vi "Exercise 5.2.vi"() -> ()   [LabVIEW 2020]
panel:
  in  "Control 2":dbl
  out "Waveform Chart 2":dbl(graph)
  in  "Master Stop":bool
  out "Waveform Chart 1":dbl(graph)
  in  "Control 1":dbl
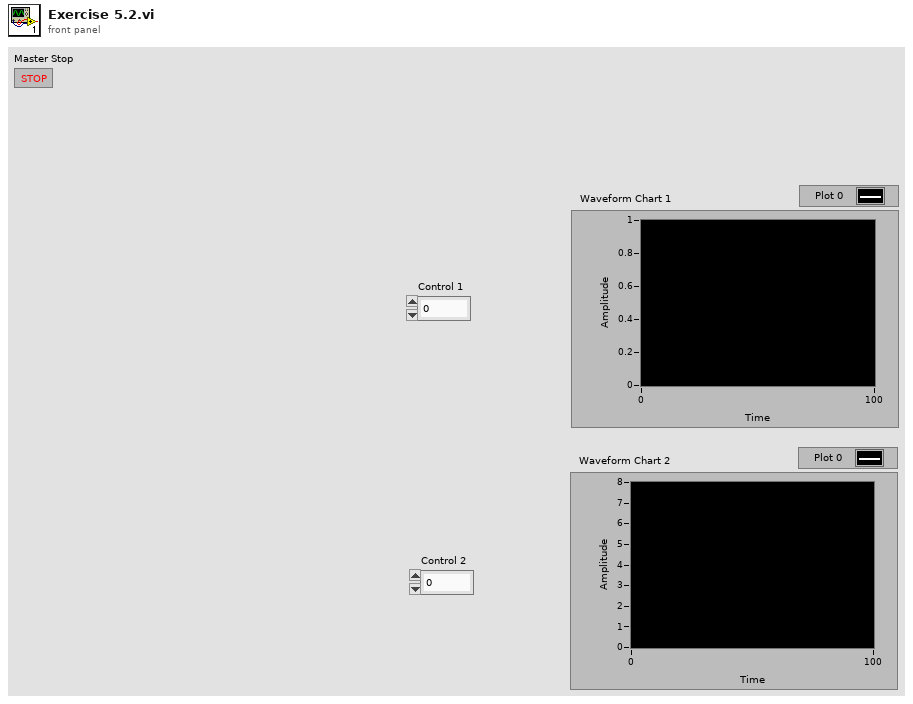
[diagram p1: front panel]
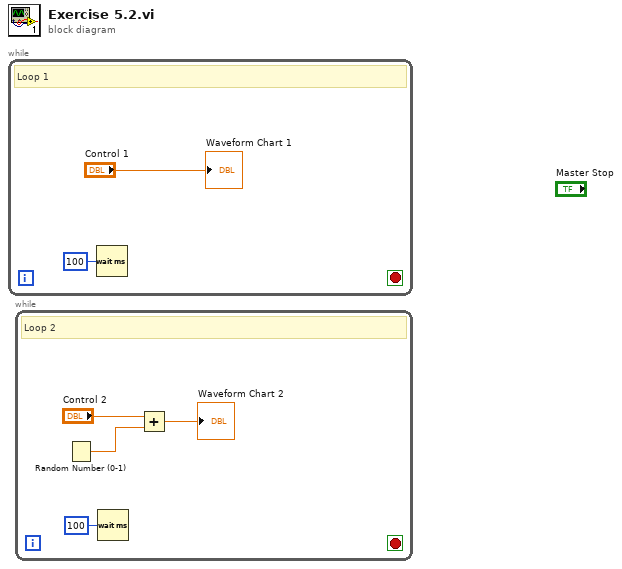
[diagram p0: block diagram]
diagram:
  n1 = while {
    stop <- _ stop-if-true
    # "Loop 1"
    n2 = Wait (ms)(milliseconds to wait=u32 100) -> ()  [unwired: 1 out]
    "Waveform Chart 1" <- "Control 1"
  }
  n3 = while {
    stop <- _ stop-if-true
    # "Loop 2"
    n4 = Random Number (0-1)() -> (number: 0 to 1=w3:dbl)
    n5 = Wait (ms)(milliseconds to wait=u32 100) -> ()  [unwired: 1 out]
    n6 = Add(x="Control 2", y=w3) -> (x+y=→"Waveform Chart 2":dbl)
  }
